vi "decimal separator.vi"() -> ()   [LabVIEW 2017]
panel:
  out "current time":timestamp format="%<%#.15X\n%x>T"
  in  "format string 4":string="%.;%<%15u>T"
  in  "format string 3":string="%,;%<%15u>T"
  out "Array 2":string[](array[string])
  in  "format string 2":string="%,;%#_16g"
  out "epsilon":ext=3.14159
  out "Array":string[](array[string])
  out "-inf":ext=3.14159
  out "+inf":ext=3.14159
  out "resulting string 2":string
  out "resulting string":string
  in  "format string":string="%.;%#_16g"
  out "input 1":ext=3.14159
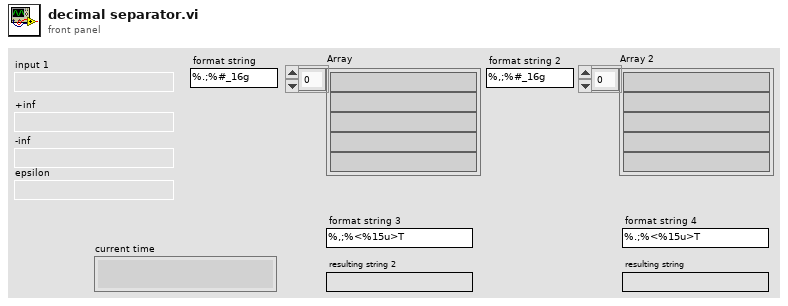
[diagram p1: front panel]
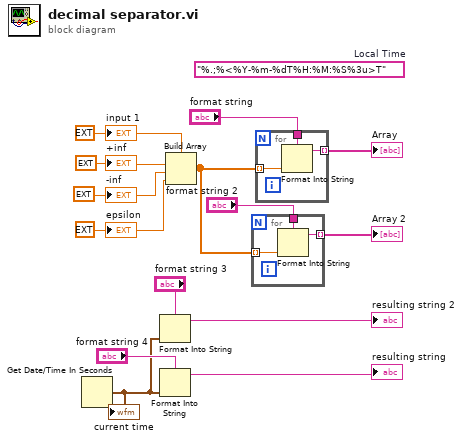
[diagram p0: block diagram]
diagram:
  w4 = ext 1.0842021724855044e-19
  w5 = ext -inf
  w6 = ext inf
  w7 = ext 3.1415926535897932385
  (unwired) "%.;%<%Y-%m-%dT%H:%M:%S%3u>T"  # Local Time
  n1 = Get Date/Time In Seconds() -> (seconds since 1Jan1904=w11:timestamp)
  "current time" <- w11
  n2 = Format Into String(format string="format string 3", w11) -> (resulting string=→"resulting string 2":string)  [unwired: 2 in, 1 out]
  n3 = Format Into String(format string="format string 4", w11) -> (resulting string=→"resulting string":string)  [unwired: 2 in, 1 out]
  n4 = Build Array(w7, w6, w5, w4) -> (w3:ext[])
  n5 = for {
    tunnel: w3 -> [w17] mode=indexing
    tunnel: "format string 2" -> [w16]
    tunnel: [w15] -> w1 mode=indexing
    n6 = Format Into String(format string=w16, w17) -> (resulting string=w15:string)  [unwired: 2 in, 1 out]
  }
  "Array 2" <- w1
  n7 = for {
    tunnel: w3 -> [w20] mode=indexing
    tunnel: "format string" -> [w19]
    tunnel: [w18] -> w8 mode=indexing
    n8 = Format Into String(format string=w19, w20) -> (resulting string=w18:string)  [unwired: 2 in, 1 out]
  }
  "Array" <- w8
  "input 1" <- w7
  "+inf" <- w6
  "-inf" <- w5
  "epsilon" <- w4
